vi "Top Coveyer Sensor.vi"(11 "Enum":enum16{"Init", "Run", "End"}(ring)=enum."Run") -> (3 "Sensor True?":bool)   [LabVIEW 2011]
uses:
  TypeDefs/Digital Module 1.ctl
  <vilib>/Rock Robotics/SystemInterfaces/Typedef/FPGA_TypedefDigitalModule.ctl
  <vilib>/Rock Robotics/SystemInterfaces/DIO/FPGA_DIOChannel.ctl
panel:
  in  "Digital Module A":T1={"Module"=enum."Digital Module 1", "Left Enc A"=enum."DIO 1", "Left Enc B"=enum."DIO 2", "Right Enc A"=enum."DIO 3", "Right Enc B"=enum."DIO 4", "Outer Sensor"=enum."DIO 5", "Inner Sensor"=enum."DIO 6", "Upper Sensor"=enum."DIO 7", "Shooter Tachometer"=enum."DIO 8", "Unassigned"=enum."DIO 9", "Unassigned"=enum."DIO 10", "Top Conveyer Sensor"=enum."DIO 11", "Arm Upper Limit"=enum."DIO 12", "Arm Lower Limit"=enum."DIO 13", "1510"=enum."DIO 14"}
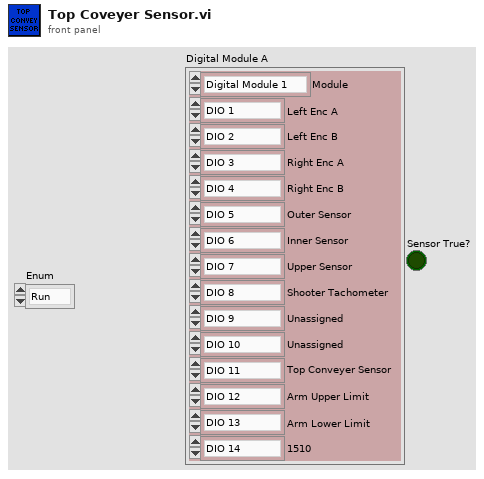
[diagram p1: front panel]
types:
  T1 = typedef "Digital Module 1.ctl" = cluster{"Module":T2, "Left Enc A":T3, "Left Enc B":T3, "Right Enc A":T3, "Right Enc B":T3, "Outer Sensor":T3, "Inner Sensor":T3, "Upper Sensor":T3, "Shooter Tachometer":T3, "Unassigned":T3, "Unassigned":T3, "Top Conveyer Sensor":T3, "Arm Upper Limit":T3, "Arm Lower Limit":T3, "1510":T3}
  T2 = typedef "FPGA_TypedefDigitalModule.ctl" = enum16{"Digital Module 1", "Digital Module 2"}
  T3 = typedef "FPGA_DIOChannel.ctl" = enum8{"DIO 1", "DIO 2", "DIO 3", "DIO 4", "DIO 5", "DIO 6", "DIO 7", "DIO 8", "DIO 9", "DIO 10", "DIO 11", "DIO 12", "DIO 13", "DIO 14", "Invalid"}
  T4 = typedef "WPI_DigitalInputDevRef.ctl" = cluster{"DevStatus":errorcluster, "DIO Channel":T3, "Digital Module":T2}
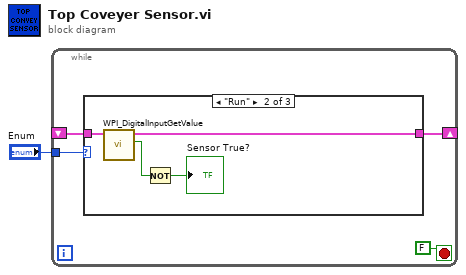
[diagram p0: block diagram]
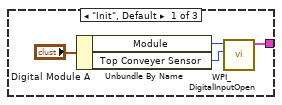
[diagram p2: hidden frame]
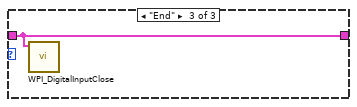
[diagram p3: hidden frame]
diagram:
  n1 = while {
    tunnel: "Enum" -> [w4]
    shift-right: [w3] -> _
    shift-left: _ -> [w2]
    stop <- FALSE stop-if-true
    n2 = case shown="\"Run\"" w4 {
      tunnel: [w6 w12 w14] -> w3
      tunnel: w2 -> [_ w13 w14]
      frame "Init", Default {
        n3 = Unbundle By Name("Digital Module A") -> ("Module"=w8:T2, "Top Conveyer Sensor"=w7:T3)
        n4 = call <vilib>:"WPI_DigitalInputOpen.vi"("DIO Channel"=w7, "Digital Module (Module 1)"=w8) -> ("DigitalInputDevRef"=w6:T4)  [unwired: 8 in, 1 out]
      }
      frame "Run" {
        n5 = call <vilib>:"WPI_DigitalInputGetValue.vi"("DigitalInputDevRef"=w13) -> ("Value"=w11:bool, "DigitalInputDevRef"=w12:T4)  [unwired: 8 in, 1 out]
        n6 = Not(x=w11) -> (.not. x?=→"Sensor True?":bool)
      }
      frame "End" {
        n7 = call <vilib>:"WPI_DigitalInputClose.vi"("DigitalInputDevRef"=w14) -> ()  [unwired: 10 in, 1 out]
      }
    }
  }
